vi "Load Test Node.vi"(8 "error in (no error)":errorcluster, 11 "Edit Test Node Model in":refnum<class "Edit Test Node Model.lvclass">) -> (0 "error out":errorcluster, 3 "Edit Test Node Model out":refnum<class "Edit Test Node Model.lvclass">)   [LabVIEW 2013, in "Edit Test Node Model.lvlib" / "Edit Test Node Model.lvclass"]
uses:
  Edit Test Node Model.lvclass
  Edit Test Node Model.lvclass/Edit Test Node Model.ctl
  Common/File IO/File IO.lvlib
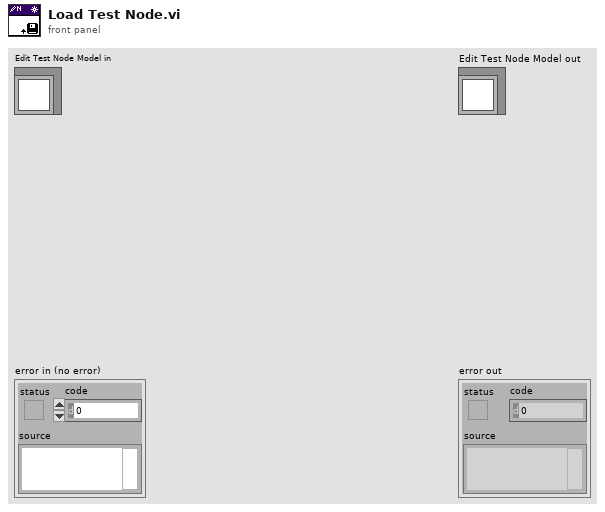
[diagram p1: front panel]
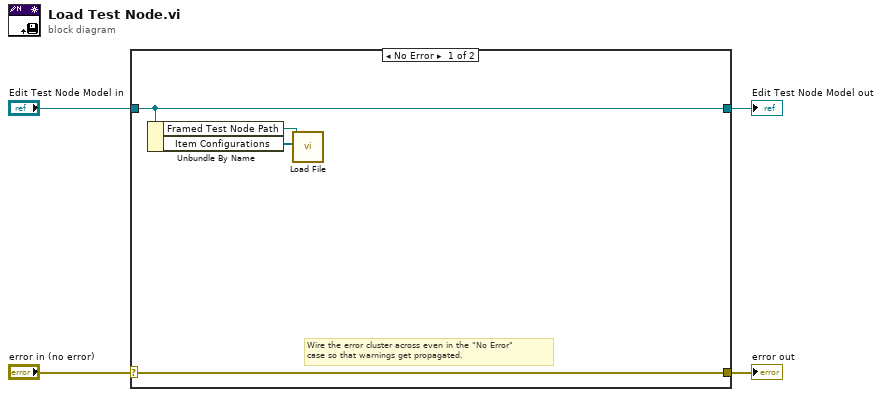
[diagram p0: block diagram]
diagram:
  n1 = case shown="No Error" "error in (no error)" {
    selector: "error in (no error)" -> [w8 w10]
    tunnel: [w8 w10] -> w3
    tunnel: [w7 w9] -> w1
    tunnel: "Edit Test Node Model in" -> [w7 w9]
    frame No Error {
      # "Wire the error cluster across even in the \"No Error\"\ncase so that warnings get propagated."
      n2 = Unbundle By Name(w7) -> ("Framed Test Node Path"=w5:path, "Item Configurations"=w6:refnum<class "Item Configuration.lvclass">[])
      n3 = call "Load File.vi"("Item Configurations"=w6, "File Path"=w5) -> ()  [unwired: 9 in, 1 out]
    }
    frame Error {
    }
  }
  "error out" <- w3
  "Edit Test Node Model out" <- w1
